vi "Interface.vi"() -> (4 "Interface":string)   [LabVIEW 2021, in "Measurement Client.lvlib"]
uses:
  Measurement Client.lvlib
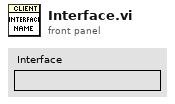
[diagram p1: front panel]
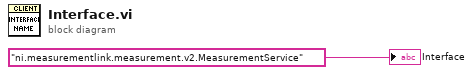
[diagram p0: block diagram]
diagram:
  "Interface" <- "ni.measurementlink.measurement.v2.MeasurementService" ("provided_interface")
